vi "Keysight 34401A Measurement Logic.vi"(8 "error in (no error)":errorcluster, 10 "session":refnum<visa-resource-name>, 11 "measurement configuration":T2) -> (0 "error out":errorcluster, 3 "measurement results":T1)   [LabVIEW 2020, in "Keysight 34401A DMM Measurement.lvlib"]
uses:
  Keysight 34401A DMM Measurement.lvlib
  Measurement Configuration.ctl
  Keysight 34401A Function.ctl
  Measurement Results.ctl
  <instrlib>/Agilent 34401/Agilent 34401.lvlib
  <instrlib>/Agilent 34401/Public/Data/Read (Single Point).vi
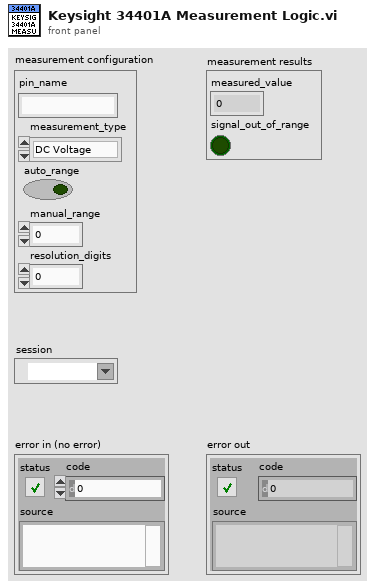
[diagram p1: front panel]
types:
  T1 = typedef "Keysight 34401A DMM Measurement.lvlib/Measurement Results.ctl" = cluster{"measured_value":dbl, "signal_out_of_range":bool}
  T2 = typedef "Keysight 34401A DMM Measurement.lvlib/Measurement Configuration.ctl" = cluster{"pin_name":string, "measurement_type":T3, "auto_range":bool, "manual_range":dbl, "resolution_digits":dbl}
  T3 = typedef "Keysight 34401A DMM Measurement.lvlib/Keysight 34401A Function.ctl" = enum16{"DC Voltage", "AC Voltage", "2 - Wire Resistance", "4 - Wire Resistance", "DC Current", "AC Current", "Frequency", "Period", "Continuity", "Diode Checking", "VDC:VDC Ratio", "Temperature", "Capacitance"}
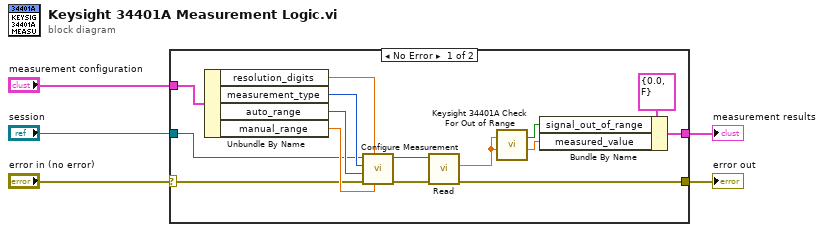
[diagram p0: block diagram]
diagram:
  n1 = case shown="No Error" "error in (no error)" {
    selector: "error in (no error)" -> [w6 w20]
    tunnel: "measurement configuration" -> [w19 _]
    tunnel: [w14 _] -> w4
    tunnel: [w13 w20] -> w3
    tunnel: "session" -> [w7 _]
    frame No Error {
      n2 = Unbundle By Name(w19) -> ("resolution_digits"=w18:dbl, "measurement_type"=w8:T3, "auto_range"=w10:bool, "manual_range"=w9:dbl)
      n3 = call <instrlib>:"Configure Measurement.vi"("Manual Range (1.00)"=w9, "Manual Resolution (5.5 Digits)"=w18, "error in (no error)"=w6, "Enable Auto Range (T: Enable)"=w10, "Function (0: DC Voltage)"=w8, "VISA resource name"=w7) -> ("error out"=w16:errorcluster, "VISA resource name out"=w17:refnum<visa-resource-name>)  [unwired: 4 in]
      n4 = call-poly <instrlib>:"Read.vi"("error in (no error)"=w16, "VISA resource name"=w17) -> ("error out"=w13:errorcluster, "Measurement"=w11:dbl)  [unwired: 7 in, 1 out]
      n5 = call "Keysight 34401A Check For Out of Range.vi"("value"=w11) -> ("out of range?"=w12:bool)  [unwired: 2 in]
      n6 = Bundle By Name(cluster=T1 {"measured_value"=0.0, "signal_out_of_range"=FALSE} ("measurement results"), "signal_out_of_range"=w12, "measured_value"=w11) -> (w14:T1)
    }
    frame Error {
    }
  }
  "measurement results" <- w4
  "error out" <- w3
